vi "Start-Stop DAQ.vi"(8 "Error In":errorcluster, 10 "Start DAQ":bool, 11 "LHW-GUI-Actor in":refnum<class "LHW-GUI-Actor.lvclass">) -> (0 "Error Out":errorcluster, 3 "LHW-GUI-Actor out":refnum<class "LHW-GUI-Actor.lvclass">)   [LabVIEW 2016, in "LHW-GUI.lvlib" / "LHW-GUI-Actor.lvclass"]
doc: "Start/Stop DAQ."
uses:
  LHW-GUI-Actor.lvclass
  LHW-GUI-Actor.lvclass/LHW-GUI-Actor.ctl
  LHW-Aquisition-Actor Messages/Start-Stop DAQ Msg/Start-Stop DAQ Msg.lvclass/Start-Stop DAQ Msg.ctl
  <vilib>/ActorFramework/Message Enqueuer/Message Enqueuer.lvclass/Message Enqueuer.ctl
  <vilib>/ActorFramework/Message Enqueuer/Enqueue.vi
  LHW-Aquisition-Actor Messages/Start-Stop DAQ Msg/Start-Stop DAQ Msg.lvclass
  C:/Program Files (x86)/National Instruments/LabVIEW 2016/vi.lib/ActorFramework/Message/Message.lvclass
  <vilib>/ActorFramework/Message Priority Queue/Priority Enqueue.vi
  <vilib>/ActorFramework/Message Enqueuer/Message Enqueuer.lvclass
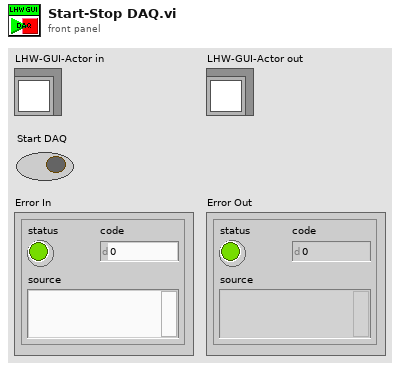
[diagram p1: front panel]
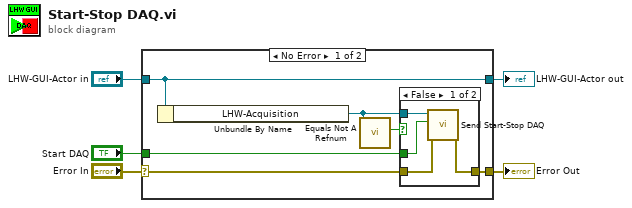
[diagram p0: block diagram]
diagram:
  n1 = case shown="No Error" "Error In" {
    selector: "Error In" -> [w9 w18]
    tunnel: [w8 w18] -> w4
    tunnel: [w11 w17] -> w2
    tunnel: "LHW-GUI-Actor in" -> [w11 w17]
    tunnel: "Start DAQ" -> [w10 _]
    frame No Error {
      n2 = Unbundle By Name(w11) -> ("LHW-Acquisition"=w7:refnum<class "Message Enqueuer.lvclass">)
      n3 = call <vilib>:"Equals Not A Refnum.vi"("Message Enqueuer"=w7) -> ("Not a refnum?"=w6:bool)  [unwired: 10 in]
      n4 = case shown="False" w6 {
        tunnel: w10 -> [w15 _]
        tunnel: w9 -> [w14 w16]
        tunnel: [w13 w16] -> w8
        tunnel: w7 -> [w12 _]
        frame False {
          n5 = call "Send Start-Stop DAQ.vi"("error in (no error)"=w14, "Start DAQ"=w15, "Message Enqueuer"=w12) -> ("error out"=w13:errorcluster)  [unwired: 7 in, 1 out]
        }
        frame True {
        }
      }
    }
    frame Error {
    }
  }
  "Error Out" <- w4
  "LHW-GUI-Actor out" <- w2
